vi "获取所有表单引用.vi"(8 "错误输入（无错误）":errorcluster, 11 "excel引用":refnum<k7>) -> (0 "错误输出":errorcluster, 2 "Worksheets":refnum<k7>, 3 "excel引用输出":refnum<k7>)   [LabVIEW 2013, in "excel处理.lvlib"]
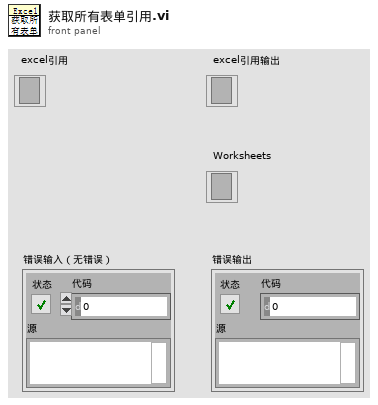
[diagram p1: front panel]
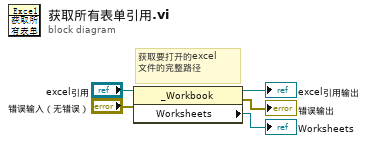
[diagram p0: block diagram]
diagram:
  # "获取要打开的excel\n文件的完整路径"
  n1 = property on="属性节点" class="_Workbook"(reference="excel引用", error in="错误输入（无错误）") -> (reference out=→"excel引用输出":refnum<k7>, error out=→"错误输出":errorcluster, "Worksheets"=→"Worksheets":refnum<k7>)
